vi "Convert Real.vi"(9 "data in":string[](array[string])) -> (1 "data out":string[](array[string]))   [LabVIEW 2018, in "LV-ORM.lvclass"]
uses:
  LV-ORM.lvclass
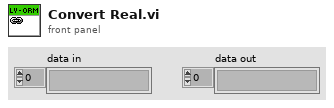
[diagram p1: front panel]
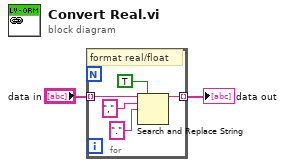
[diagram p0: block diagram]
diagram:
  n1 = for {
    tunnel: "data in" -> [w5] mode=indexing
    tunnel: [w4] -> w1 mode=indexing
    # "format real/float"
    n2 = Search and Replace String(replace all?=TRUE, input string=w5, search string=",", replace string=".") -> (result string=w4:string)  [unwired: 4 in, 3 out]
  }
  "data out" <- w1
